vi "1 byte transfer.vi"(1 "Min time SCL low (uSec)":u32, 2 "Min Time SCL high (uSec)":u32, 3 "Data bit array":bool[](array[boolean])) -> ()   [LabVIEW 2013]
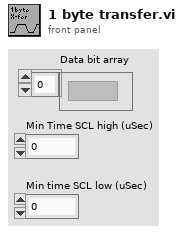
[diagram p1: front panel]
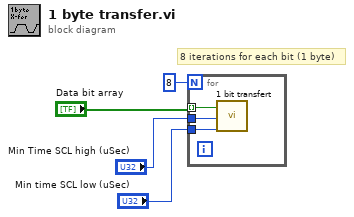
[diagram p0: block diagram]
diagram:
  # "8 iterations for each bit (1 byte)"
  n1 = for {
    N: 8 -> [_]
    tunnel: "Min Time SCL high (uSec)" -> [w6]
    tunnel: "Min time SCL low (uSec)" -> [w7]
    tunnel: "Data bit array" -> [w5] mode=indexing
    n2 = call "1 bit transfert.vi"("Min time SCL low (uSec)"=w7, "Min Time SCL high (uSec)"=w6, "Data bit"=w5) -> ()  [unwired: 1 in]
  }
